vi "Choreo_TrajectoryState_GetAll.vi"(11 "ChoreoTrajectoryState":T1) -> (0 "velocityX":dbl, 1 "heading":dbl, 2 "y":dbl, 3 "x":dbl, 4 "velocityY":dbl, 5 "timestamp":dbl, 6 "angularVelocity":dbl)   [LabVIEW 2019, in "ChoreoLib.lvlib"]
doc: "Return individual data from a ChoreoTrajectoryState cluster\n\nInputs:\n - ChoreoTrajectoryState - cluster - Individual trajectory state\n\nOutputs: \n - timestamp - double - The timestamp of this state, relative to the beginning of the trajectory.\n - x - double - The X position of the state in meters. \n - y - double - The Y position of the state in meters.\n - heading - double - The heading of the state in radians, with 0 being in the +X direction.\n - velocityX - double - The velocity of the state in the X direction in m/s.\n - velocityY - double - The velocity of the state in the X direction in m/s.\n - angularVelocity - double - The angular velocity of the state in rad/s."
uses:
  ChoreoLib.lvlib
  TypeDef/ChoreoTrajectoryState.ctl
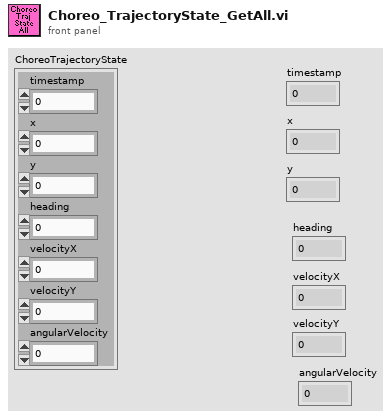
[diagram p1: front panel]
types:
  T1 = typedef "ChoreoLib.lvlib/ChoreoTrajectoryState.ctl" = cluster{"timestamp":dbl, "x":dbl, "y":dbl, "heading":dbl, "velocityX":dbl, "velocityY":dbl, "angularVelocity":dbl}
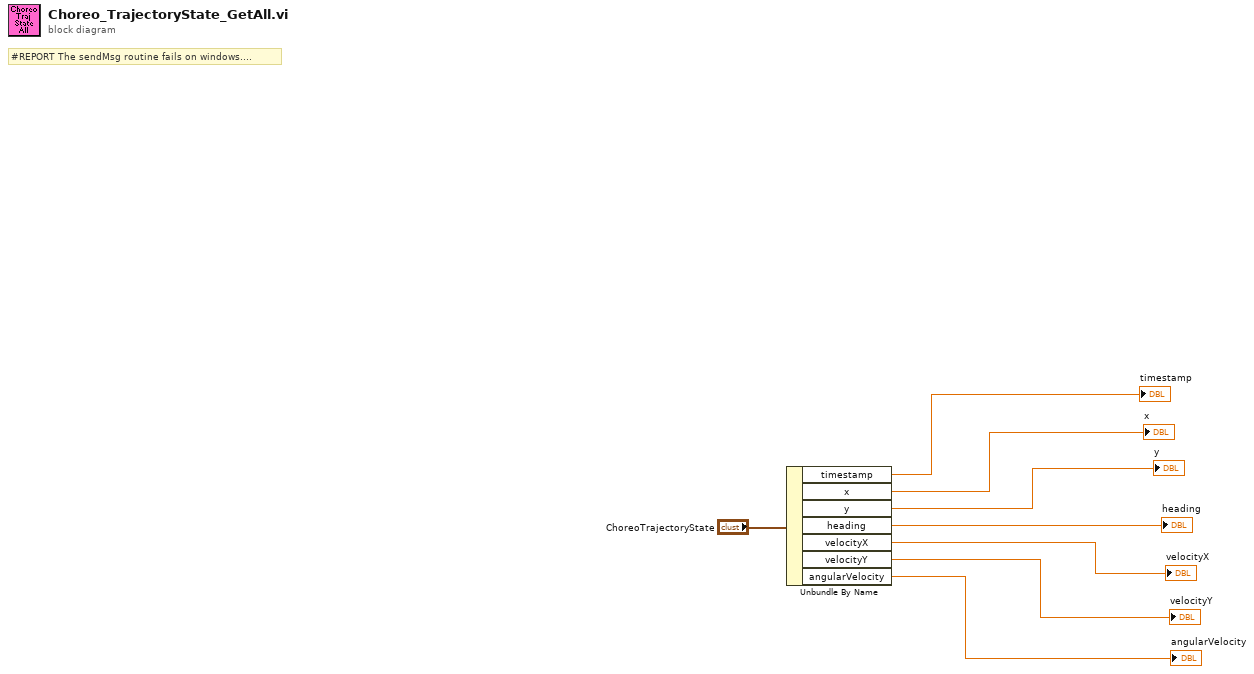
[diagram p0: block diagram]
diagram:
  # "#REPORT The sendMsg routine fails on windows...."
  n1 = Unbundle By Name("ChoreoTrajectoryState") -> ("timestamp"=→"timestamp":dbl, "x"=→"x":dbl, "y"=→"y":dbl, "heading"=→"heading":dbl, "velocityX"=→"velocityX":dbl, "velocityY"=→"velocityY":dbl, "angularVelocity"=→"angularVelocity":dbl)
